vi "Autonomous Independent.vi"() -> ()   [LabVIEW 2017]
doc: "This VI is called when autonomous begins, and will automatically be terminated when autonomous ends. You can carry out timed or sensor driven robot movement independently without needing to return to the caller."
uses:
  <vilib>/Rock Robotics/WPI/ThirdParty/Phoenix-LabVIEW/Motor Controller/Controls/CTRE_Phoenix_MotorControl_ControlMode.ctl
  <vilib>/Rock Robotics/WPI/Utilities/WPI_GetSetVariantRefNum.vi
  <vilib>/Rock Robotics/Network Tables/NT Read String.vi
  <vilib>/Rock Robotics/Network Tables/NT Write Numeric Array.vi
  <vilib>/Rock Robotics/Network Tables/NT Read Number.vi
  Robot Global Data.vi
panel:
  in  "P 3":dbl=1.0
  in  "PhaseSensor 2":bool
  in  "PhaseSensor":bool
  in  "I Zone 2":dbl
  in  "F 2":dbl
  in  "D 2":dbl=0.001
  in  "I 2":dbl
  in  "P 2":dbl=1.0
  in  "I Zone":dbl
  in  "F":dbl
  # "Be sure to right-click and choose Data Operations>>Make Current Value default if you want to save the array values with the VI"
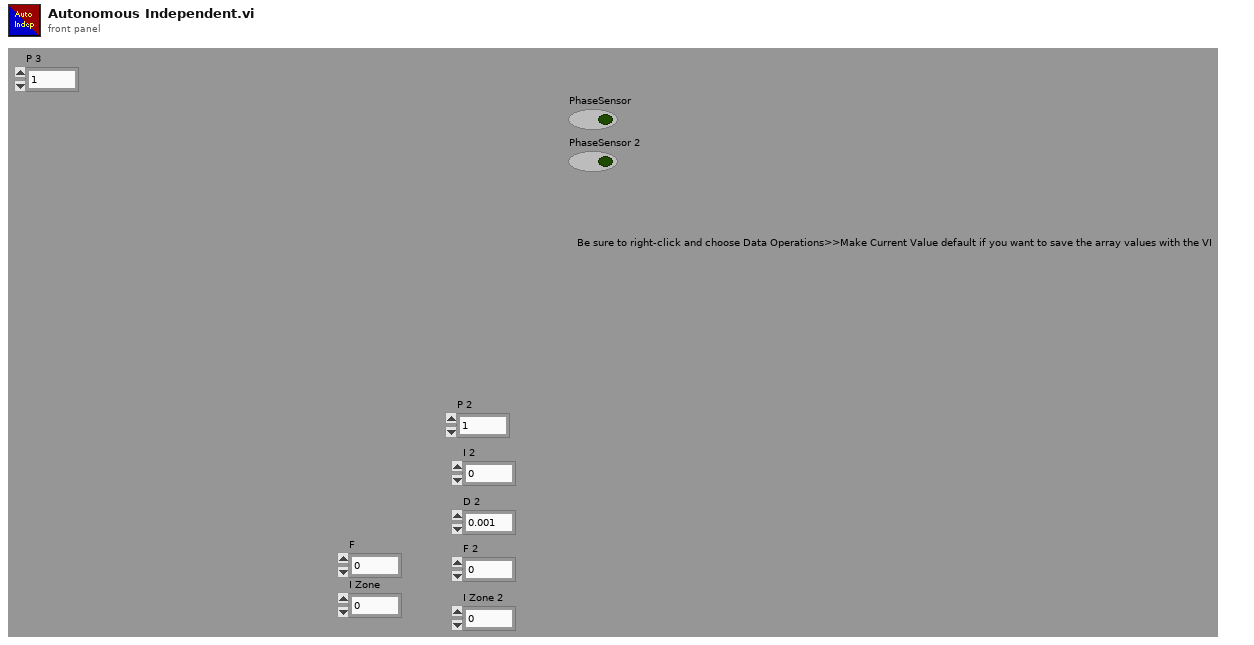
[diagram p1: front panel]
types:
  T1 = typedef "WPI_JoystickDevRef.ctl" = cluster{"Device":T2}
  T2 = typedef "WPI_JoystickDeviceEnum.ctl" = enum16{"USB 0", "USB 1", "USB 2", "USB 3", "USB 4", "USB 5"}
  T3 = cluster{"Yaw":dbl, "Roll":dbl, "Pitch":dbl, "Heading":dbl, "Fused Heading":dbl}
  T4 = typedef "WPI_MotorControlDeviceRef.ctl" = cluster{"DeviceStatus":errorcluster, "Type":T5, "PWM":cluster{"PWM Channel":T6, "DeadBand":T7}, "CAN":cluster{"Device Number":u8, "SetOutput VI Ref":variant, "GetOutput VI Ref":variant, "Enable VI Ref":variant, "Disable VI Ref":variant, "Data":variant}, "Invert":bool, "DIO PWM":cluster{"PWM \"Enable\" Channel":T6, "DIOChannel":T8, "PWM Rate":dbl}}
  T5 = typedef "WPI_MotorControlType.ctl" = enum16{"PWM", "CAN", "DIO PWM"}
  T6 = typedef "FPGA_DIOPWMChannel.ctl" = enum8{"PWM 0", "PWM 1", "PWM 2", "PWM 3", "PWM 4", "PWM 5", "PWM 6", "PWM 7", "PWM 8", "PWM 9", "PWM MXP 0", "PWM MXP 1", "PWM MXP 2", "PWM MXP 3", "PWM MXP 4", "PWM MXP 5", "PWM MXP 6", "PWM MXP 7", "PWM MXP 8", "PWM MXP 9", "Invalid"}
  T7 = typedef "WPI_PWMDeadband.ctl" = cluster{"Name":string, "maxPositivePwm":i32, "minPositivePwm":i32, "centerPwm":i32, "maxNegativePwm":i32, "minNegativePwm":i32, "angularRange":u16}
  T8 = typedef "FPGA_DIOChannel.ctl" = enum8{"DIO 0", "DIO 1", "DIO 2", "DIO 3", "DIO 4", "DIO 5", "DIO 6", "DIO 7", "DIO 8", "DIO 9", "DIO MXP 0", "DIO MXP 1", "DIO MXP 2", "DIO MXP 3", "DIO MXP 4", "DIO MXP 5", "DIO MXP 6", "DIO MXP 7", "DIO MXP 8", "DIO MXP 9", "DIO MXP 10", "DIO MXP 11", "DIO MXP 12", "DIO MXP 13", "DIO MXP 14", "DIO MXP 15", "SPI Port CS1", "SPI Port CS2", "SPI Port CS3", "SPI Port MISO", "SPI Port MOSI", "Invalid"}
  T9 = typedef "CTRE_Phoenix_MotorControl_ControlMode.ctl" = u16
  T10 = typedef "WPI_RobotDriveDevRef.ctl" = cluster{"DevStatus":errorcluster, "Motors[]":T4[], "Square Inputs":bool, "Max Output":dbl}
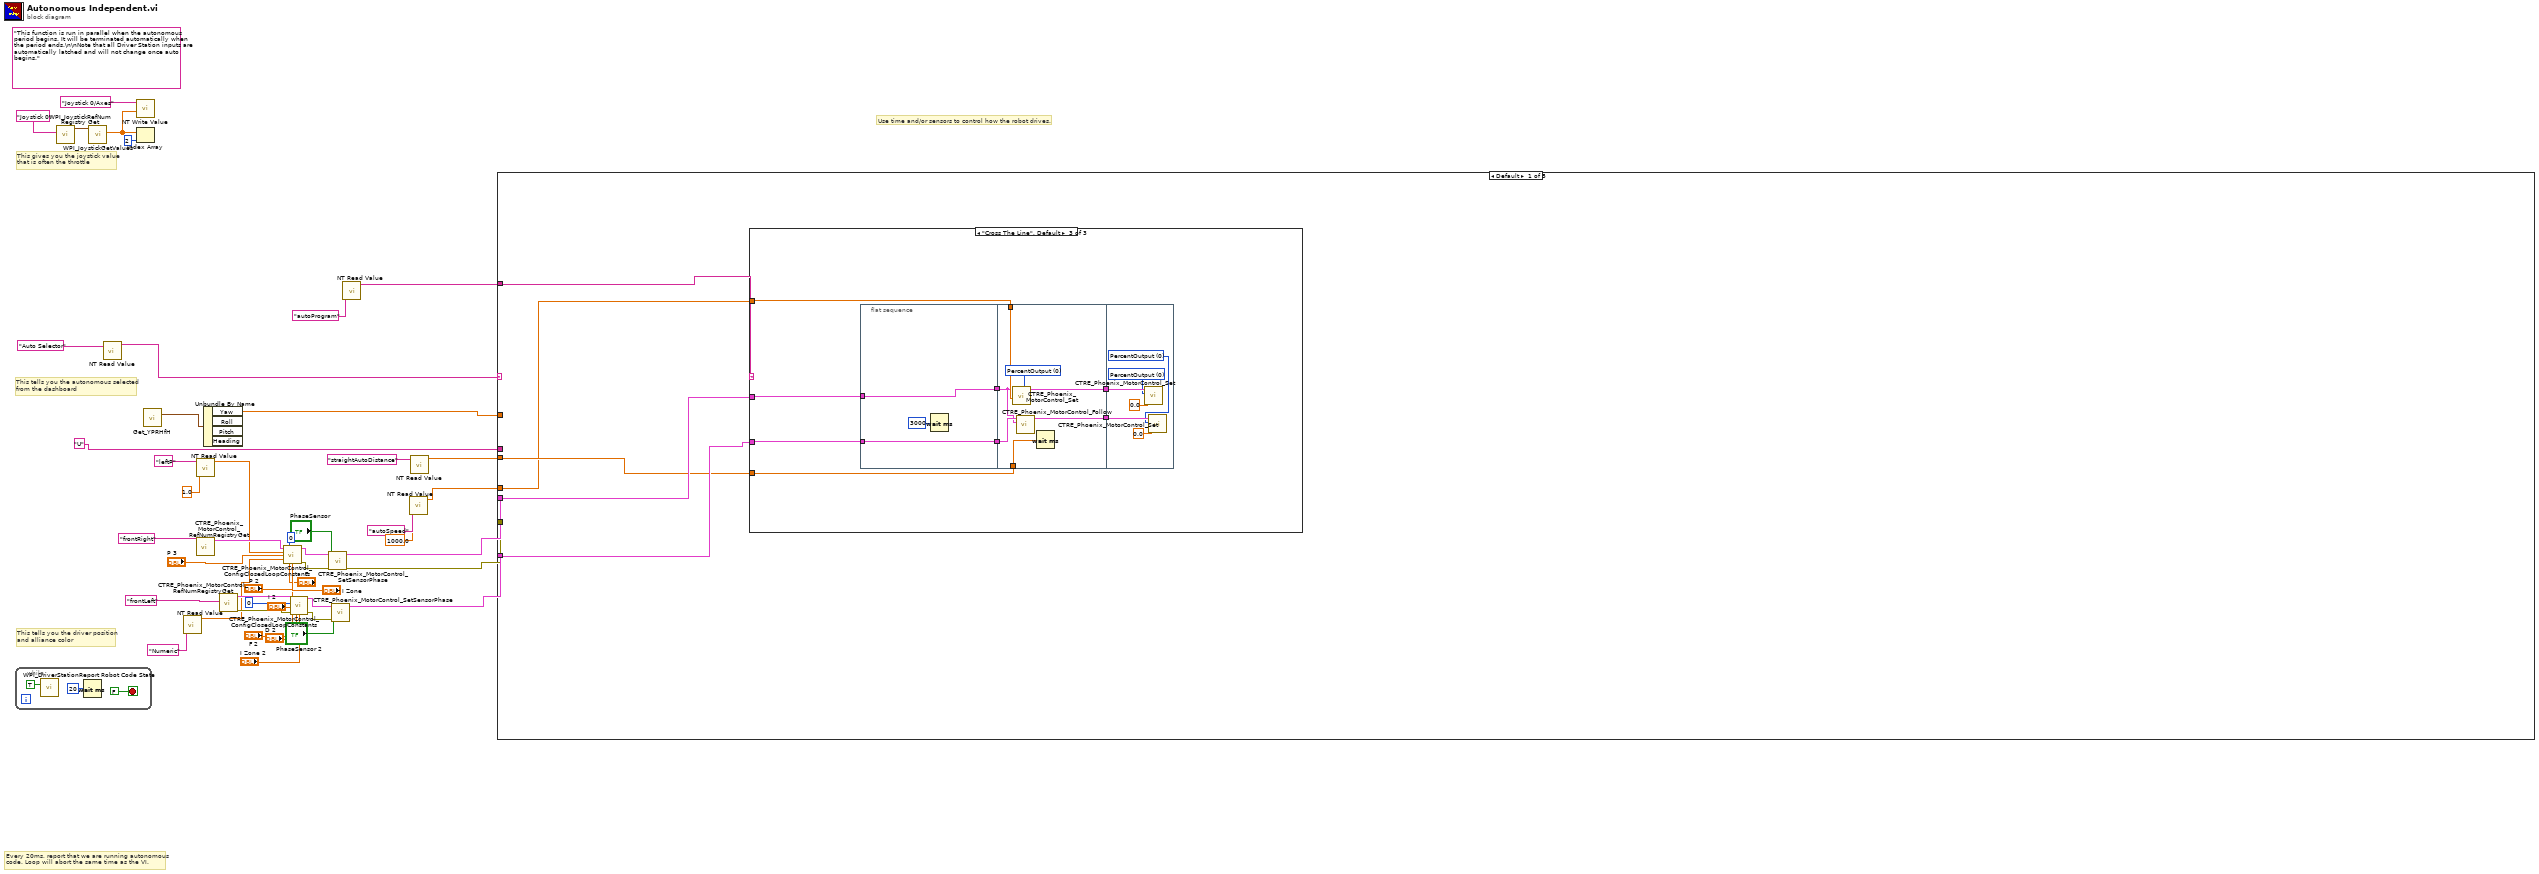
[diagram p0: block diagram]
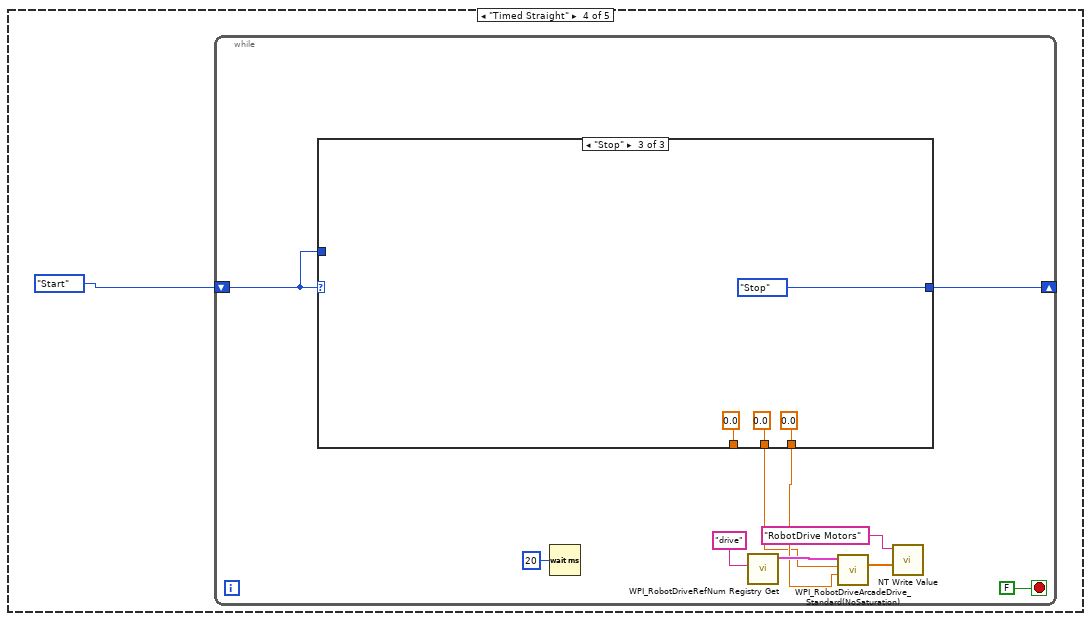
[diagram p6: hidden frame]
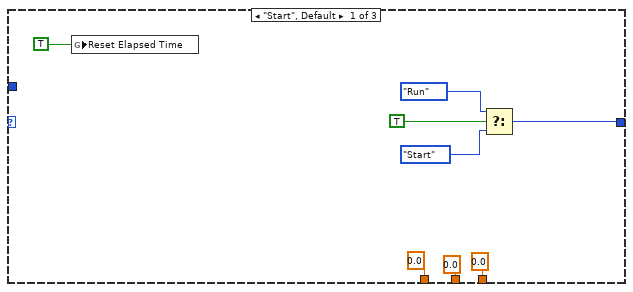
[diagram p7: hidden frame]
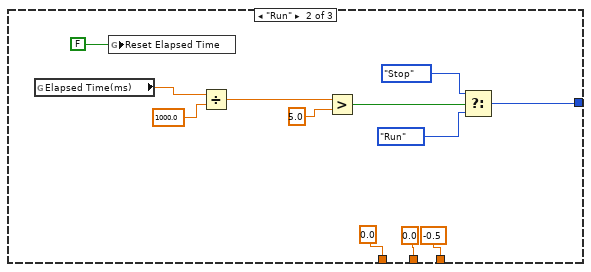
[diagram p8: hidden frame]
diagram:
  (unwired) "This function is run in parallel when the autonomous period begins. It will be terminated automatically when the period ends.\n\nNote that all Driver Station inputs are automatically latched and will not change once auto begins."
  # "This tells you the autonomous selected\nfrom the dashboard"
  # "Every 20ms, report that we are running autonomous\ncode. Loop will abort the same time as the VI."
  # "This gives you the joystick value\nthat is often the throttle"
  # "Use time and/or sensors to control how the robot drives."
  # "This tells you the driver position\nand alliance color"
  n1 = while {
    stop <- FALSE stop-if-true
    n2 = call <vilib>:"WPI_DriverStationReport Robot Code State.vi"("Autonomous"=TRUE) -> ()  [unwired: 10 in, 1 out]
    n3 = Wait (ms)(milliseconds to wait=u32 20) -> ()  [unwired: 1 out]
  }
  n4 = call <vilib>:"WPI_JoystickRefNum Registry Get.vi"("refnum name"="Joystick 0") -> ("JoystickDevRef"=w45:T1)  [unwired: 1 in, 9 out]
  n5 = call <vilib>:"WPI_JoystickGetValues.vi"("JoystickDevRef"=w45) -> ("Axes"=w41:dbl[])  [unwired: 6 in, 4 out]
  n6 = call-poly <vilib>:"NT Read Value.vi"("Name"="Auto Selector") -> ("String"=w42:string)  [unwired: 9 in, 1 out]
  n7 = call-poly <vilib>:"NT Write Value.vi"("Numeric Array"=w41, "Name"="Joystick 0/Axes") -> ()  [unwired: 9 in, 1 out]
  n8 = Index Array(array=w41, index=2) -> ()  [unwired: 1 out]
  n9 = call <vilib>:"Get_YPRHfH.vi"() -> ("YRPHfH"=w38:T3)  [unwired: 11 in]
  n10 = call-poly <vilib>:"NT Read Value.vi"("Name"="Numeric") -> ("Numeric"=w9:dbl)  [unwired: 9 in, 1 out]
  n11 = call <vilib>:"CTRE_Phoenix_MotorControl_RefNumRegistryGet.vi"("refnum name"="frontRight") -> ("PhoenixMotorControlDevRef"=w32:T4)  [unwired: 9 in, 1 out]
  n12 = call-poly <vilib>:"NT Read Value.vi"("Default Value"=1.0, "Name"="leftP") -> ("Numeric"=w10:dbl)  [unwired: 8 in, 1 out]
  n13 = Unbundle By Name(w38) -> ("Yaw"=w37:dbl)  [unwired: 3 out]
  n14 = call <vilib>:"CTRE_Phoenix_MotorControl_RefNumRegistryGet.vi"("refnum name"="frontLeft") -> ("error out"=w29:errorcluster, "PhoenixMotorControlDevRef"=w30:T4)  [unwired: 9 in]
  n15 = call <vilib>:"CTRE_Phoenix_MotorControl_ConfigClosedLoopConstants.vi"("PhoenixMotorControlDevRef"=w32, "slotIdx"=0, "P"=w10, "I"="P 3", "D"=w9, "F"="F", "I Zone"="I Zone") -> ("PhoenixMotorControlDevRef"=w20:T4, "error out"=w19:errorcluster)  [unwired: 7 in]
  n16 = call <vilib>:"CTRE_Phoenix_MotorControl_ConfigClosedLoopConstants.vi"("PhoenixMotorControlDevRef"=w30, "slotIdx"=0, "P"="P 2", "I"="I 2", "D"="D 2", "error in (no error)"=w29, "F"="F 2", "I Zone"="I Zone 2") -> ("PhoenixMotorControlDevRef"=w23:T4, "error out"=w22:errorcluster)  [unwired: 6 in]
  n17 = call <vilib>:"CTRE_Phoenix_MotorControl_SetSensorPhase.vi"("error in (no error)"=w19, "PhaseSensor"="PhaseSensor", "PhoenixMotorControlDevRef"=w20) -> ("error out"=w17:errorcluster, "PhoenixMotorControlDevRef"=w18:T4)  [unwired: 7 in]
  n18 = call <vilib>:"CTRE_Phoenix_MotorControl_SetSensorPhase.vi"("error in (no error)"=w22, "PhaseSensor"="PhaseSensor 2", "PhoenixMotorControlDevRef"=w23) -> ("PhoenixMotorControlDevRef"=w21:T4)  [unwired: 7 in, 1 out]
  n19 = call-poly <vilib>:"NT Read Value.vi"("Name"="autoProgram") -> ("String"=w6:string)  [unwired: 9 in, 1 out]
  n20 = call-poly <vilib>:"NT Read Value.vi"("Default Value"=1000.0, "Name"="autoSpeed") -> ("Numeric"=w2:dbl)  [unwired: 8 in, 1 out]
  n21 = call-poly <vilib>:"NT Read Value.vi"("Name"="straightAutoDistance") -> ("Numeric"=w4:dbl)  [unwired: 9 in, 1 out]
  n22 = case shown="Default" w42 {
    tunnel: "U" -> [_ _ _ _ _]
    tunnel: w37 -> [_ _ _ _ _]
    tunnel: w21 -> [w52 _ _ _ _]
    tunnel: w18 -> [w53 _ _ _ _]
    tunnel: w17 -> [_ _ _ _ _]
    tunnel: w6 -> [w54 _ _ _ _]
    tunnel: w4 -> [w51 _ _ _ _]
    tunnel: w2 -> [w50 _ _ _ _]
    frame Default {
      n23 = case shown="\"Cross The Line\", Default" w54 {
        tunnel: w53 -> [_ _ w55]
        tunnel: w52 -> [_ _ w56]
        tunnel: w51 -> [_ _ w57]
        tunnel: w50 -> [_ _ w58]
        frame "Deliver A Cube" {
        }
        frame "Do Nothing" {
        }
        frame "Cross The Line", Default {
          n24 = flat-sequence {
            tunnel: [w64] -> w62
            tunnel: w55 -> [w64]
            tunnel: [w63] -> w61
            tunnel: w56 -> [w63]
            tunnel: w62 -> [w68]
            tunnel: w61 -> [w69]
            tunnel: w57 -> [w70]
            tunnel: w58 -> [w72]
            tunnel: [w67] -> w60
            tunnel: [w66] -> w59
            tunnel: w60 -> [w78]
            tunnel: w59 -> [w74]
            frame #0 {
              n25 = Wait (ms)(milliseconds to wait=u32 3000) -> ()  [unwired: 1 out]
            }
            frame #1 {
              w71 = T9 0 items=["PercentOutput"=0, "Position"=1, "Velocity"=2, "Current"=3, "Follower"=5, "MotionProfile"=6, "MotionMagic"=7, "MotionMagicArc"=8, "MotionProfileArc"=10, "Disabled"=15] ("Control Mode")
              n26 = call <vilib>:"CTRE_Phoenix_MotorControl_Set.vi"("Output"=w72, "Control Mode"=w71, "PhoenixMotorControlDevRef"=w68) -> ("PhoenixMotorControlDevRef"=w67:T4)  [unwired: 7 in, 1 out]
              n27 = call <vilib>:"CTRE_Phoenix_MotorControl_Follow.vi"("Master Controller to Follow"=w68, "PhoenixMotorControlDevRef"=w69) -> ("PhoenixMotorControlDevRef"=w66:T4)  [unwired: 8 in, 1 out]
              n28 = Wait (ms)(milliseconds to wait=w70) -> ()  [unwired: 1 out]
            }
            frame #2 {
              w73 = T9 0 items=["PercentOutput"=0, "Position"=1, "Velocity"=2, "Current"=3, "Follower"=5, "MotionProfile"=6, "MotionMagic"=7, "MotionMagicArc"=8, "MotionProfileArc"=10, "Disabled"=15] ("Control Mode")
              w77 = T9 0 items=["PercentOutput"=0, "Position"=1, "Velocity"=2, "Current"=3, "Follower"=5, "MotionProfile"=6, "MotionMagic"=7, "MotionMagicArc"=8, "MotionProfileArc"=10, "Disabled"=15] ("Control Mode")
              n29 = call <vilib>:"CTRE_Phoenix_MotorControl_Set.vi"("Output"=0.0, "Control Mode"=w77, "PhoenixMotorControlDevRef"=w78) -> ()  [unwired: 7 in, 2 out]
              n30 = call <vilib>:"CTRE_Phoenix_MotorControl_Set.vi"("Output"=0.0, "Control Mode"=w73, "PhoenixMotorControlDevRef"=w74) -> ()  [unwired: 7 in, 2 out]
            }
          }
        }
      }
    }
    frame "Alternative 1" {
    }
    frame "Alternative 2" {
    }
    frame "Timed Straight" {
      n31 = while {
        shift-right: [w89] -> _
        shift-left: enum16{"Start", "Run", "Stop"}."Start" ("Enum") -> [w88]
        stop <- FALSE stop-if-true
        n32 = case shown="\"Stop\"" w88 {
          tunnel: [0.0 ("X") 0.0 ("X") 0.0 ("X")] -> _
          tunnel: [0.0 ("X") 0.0 ("X") 0.0 ("X")] -> w80
          tunnel: [0.0 ("X") -0.5 ("X") 0.0 ("X")] -> w81
          tunnel: [w91 w104 enum16{"Start", "Run", "Stop"}."Stop" ("Enum")] -> w89
          tunnel: w88 -> [_ _ _]
          frame "Start", Default {
            n33 = global write "Robot Global Data.vi" "Reset Elapsed Time"(TRUE ("Reset Elapsed Time")) -> ()
            n34 = Select(t=enum16{"Start", "Run", "Stop"}."Run" ("Enum"), s=TRUE, f=enum16{"Start", "Run", "Stop"}."Start" ("Enum")) -> (s? t:f=w91:enum16{"Start", "Run", "Stop"})
          }
          frame "Run" {
            n35 = global read "Robot Global Data.vi" "Elapsed Time(ms)"() -> (w102:dbl)
            n36 = global write "Robot Global Data.vi" "Reset Elapsed Time"(FALSE ("Reset Elapsed Time")) -> ()
            n37 = Divide(x=w102, y=1000.0) -> (x/y=w103:dbl)
            n38 = Greater?(x=w103, y=5.0) -> (0:w99:bool)
            n39 = Select(t=enum16{"Start", "Run", "Stop"}."Stop" ("Enum"), s=w99, f=enum16{"Start", "Run", "Stop"}."Run" ("Enum")) -> (s? t:f=w104:enum16{"Start", "Run", "Stop"})
          }
          frame "Stop" {
          }
        }
        n40 = Wait (ms)(milliseconds to wait=u32 20) -> ()  [unwired: 1 out]
        n41 = call <vilib>:"WPI_RobotDriveRefNum Registry Get.vi"("refnum name"="drive") -> ("RobotDriveDevRef"=w84:T10)  [unwired: 1 in, 9 out]
        n42 = call <vilib>:"WPI_RobotDriveArcadeDrive_Standard(NoSaturation).vi"("Y axis value"=w81, "X axis value"=w80, "RobotDriveDevRef"=w84) -> ("Motor Values"=w83:dbl[])  [unwired: 1 in, 7 out]
        n43 = call-poly <vilib>:"NT Write Value.vi"("Numeric Array"=w83, "Name"="RobotDrive Motors") -> ()  [unwired: 9 in, 1 out]
      }
    }
    frame "Your Turn" {
    }
  }
